vi "更改表格背景颜色.vi"(0 "NI_report输入":refnum<class "NI_report.lvclass">, 5 "表格":string[][](array[string]), 9 "单个结果":bool[][](array[boolean]), 11 "错误输入（无错误）":errorcluster, 12 "MS Office parameters out":T1) -> (4 "NI_report输出":refnum<class "NI_report.lvclass">, 15 "错误输出":errorcluster)   [LabVIEW 2014]
uses:
  <vilib>/Utility/NIReport.llb/NI_report.lvclass
  <vilib>/Utility/NIReport.llb/Excel/NI_Excel.lvclass
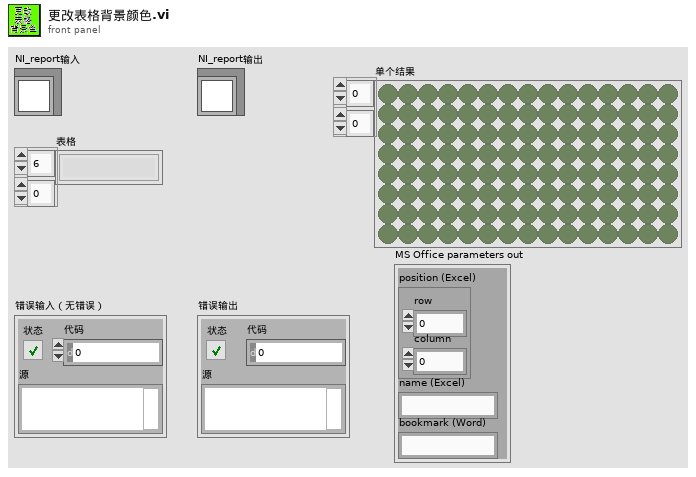
[diagram p1: front panel]
types:
  T1 = cluster{"position (Excel)":cluster{"row":i32, "column":i32}, "name (Excel)":string, "bookmark (Word)":string}
  T2 = cluster{"on/off":bool, "weight":i32, "color":u32}
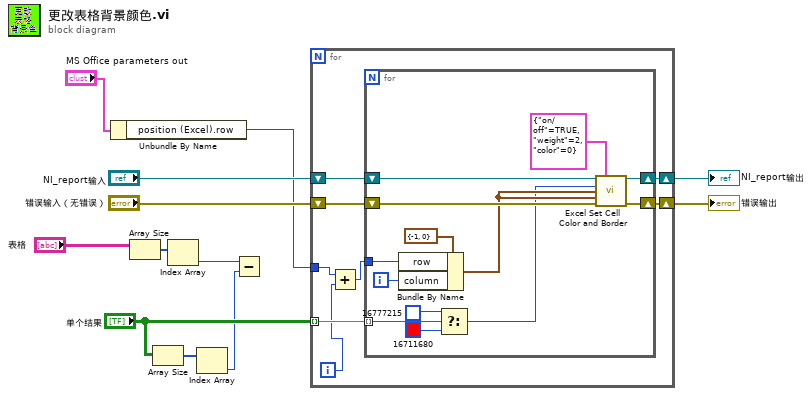
[diagram p0: block diagram]
diagram:
  n1 = Unbundle By Name("MS Office parameters out") -> ("position (Excel).row"=w1:i32)
  n2 = Array Size(array="表格") -> (size(s)=w7:i32[])
  n3 = Array Size(array="单个结果") -> (size(s)=w5:i32[])
  n4 = Index Array(array=w7) -> (element=w3:i32)  [unwired: 1 in]
  n5 = Index Array(array=w5) -> (element=w4:i32)  [unwired: 1 in]
  n6 = Subtract(x=w3, y=w4) -> ()  [unwired: 1 out]
  n7 = for {
    tunnel: w1 -> [w15]
    tunnel: "单个结果" -> [w16] mode=indexing
    shift-right: [w20] -> w12
    shift-left: "错误输入（无错误）" -> [w19]
    shift-right: [w18] -> w9
    shift-left: "NI_report输入" -> [w17]
    i -> [w14]
    n8 = Add(x=w15, y=w14) -> (x+y=w13:i32)
    n9 = for {
      tunnel: w13 -> [w26]
      shift-right: [w33] -> w20
      shift-left: w19 -> [w32]
      shift-right: [w31] -> w18
      shift-left: w17 -> [w30]
      tunnel: w16 -> [w23] mode=indexing
      i -> [w21]
      n10 = Bundle By Name(cluster=cluster{"row":i32, "column":i32} {"row"=-1, "column"=0} ("start (-1, -1)"), "row"=w26, "column"=w21) -> (w28:cluster{"row":i32, "column":i32})
      n11 = Select(t=u32 16777215 ("background color (w)"), s=w23, f=u32 16711680 ("background color (w)")) -> (s? t:f=w22:u32)
      n12 = call <vilib>:"Excel Set Cell Color and Border.vi"("report in"=w30, "inside border"=T2 {"on/off"=TRUE, "weight"=2, "color"=0}, "background color (w)"=w22, "start (-1, -1)"=w28, "end (-1, -1)"=w28, "error in (no error)"=w32) -> ("report out"=w31:refnum<class "NI_report.lvclass">, "error out"=w33:errorcluster)  [unwired: 8 in]
    }
  }
  "错误输出" <- w12
  "NI_report输出" <- w9
